vi "SetClassCtrl.vi"(8 "error in (no error)":errorcluster caption="entrée d'erreur (pas d'erreur)", 10 "ClassCtrlRef":refnum<vi>, 11 "Tools en entrée":refnum<class "Tools.lvclass"> caption="DNL_LabVIEW Object in") -> (0 "error out":errorcluster caption="sortie d'erreur", 3 "Tools en sortie":refnum<class "Tools.lvclass"> caption="DNL_LabVIEW Object out")   [LabVIEW 2019, in "Tools.lvclass"]
uses:
  Tools.lvclass
  BaseDevice/BaseDevice.lvclass
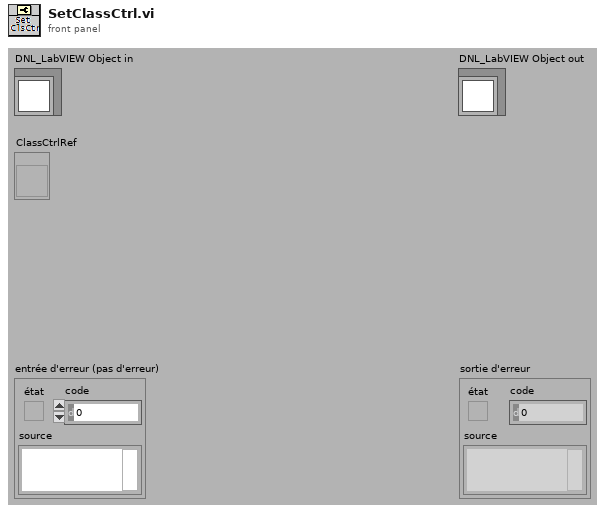
[diagram p1: front panel]
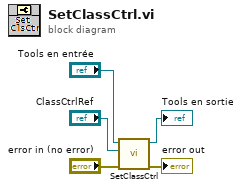
[diagram p0: block diagram]
diagram:
  n1 = call-parent "SetClassCtrl.vi"("error in (no error)"="error in (no error)", "ClassCtrlRef"="ClassCtrlRef", "BaseDevice en entrée"="Tools en entrée") -> ("error out"=→"error out":errorcluster, "BaseDevice en sortie"=→"Tools en sortie":refnum<class "Tools.lvclass">)  [unwired: 7 in]
